vi "InjA-Image-FPGA.vi"() -> ()   [LabVIEW 2016]
uses:
  Common-Control/Glassman Readback.ctl
  Common-Control/Gate Valve Readback.ctl
  Common-Control/Faraday Cup Readback.ctl
  Common-Control/Aperture Readback.ctl
  Common-Control/Glassman Control.ctl
  <vilib>/LabVIEW Targets/FPGA/cRIO/shared/nicrio_ModuleControls/nicrio_cRIO-9871_DataBitsEnum.ctl
  <vilib>/LabVIEW Targets/FPGA/cRIO/shared/nicrio_ModuleControls/nicrio_cRIO-9871_BaudRateEnum.ctl
  <vilib>/LabVIEW Targets/FPGA/cRIO/shared/nicrio_ModuleControls/nicrio_cRIO-9871_ParityEnum.ctl
  <vilib>/LabVIEW Targets/FPGA/cRIO/shared/nicrio_ModuleControls/nicrio_cRIO-9871_StopBitsEnum.ctl
  <vilib>/Platform/TimedLoop/XDataNode/timing_clust.ctl
  <vilib>/Platform/TimedLoop/XDataNode/nitl_modes.ctl
  <vilib>/Platform/TimedLoop/XDataNode/wakeup.ctl
  <vilib>/rvi/FXPMathLib/basic elements/FxpIntAccumulator/subVIs/nifxpmath_IntAccumulator_SimConfig.ctl
  <vilib>/rvi/Emulation/niFpgaGetClockAttributes.vi
  <vilib>/rvi/Emulation/niFpgaSctlEmulationGetInTimedLoop.vi
  <vilib>/rvi/Emulation/niFpgaEmulationReportErrorSimple.vi
  <vilib>/rvi/eio/common/nirviEmuTemplateMethod_errors.vi
  <vilib>/rvi/Emulation/niFpgaCriticalErrorInLSC.vi
  <vilib>/rvi/Analysis/common/codeGenErrors/XNode/niFpgaXNodeCodeGenErrorHandle.vi
  <vilib>/rvi/FXPMathLib/basic elements/FxpIntAccumulator/simVIs/DllFxpIntAccumulator_sub.vi
  <vilib>/rvi/eio/common/nirviEmuTemplatePropertySet_errors.vi
  <vilib>/eio/EIONode/EIONode.xnode
  <vilib>/rvi/Analysis/measure/dc-rms/XNode/niFpgaDC-RMS.xnode
  <vilib>/Platform/TimedLoop/XDataNode/XDataNode.xnode
  <vilib>/rvi/FXPMathLib/basic elements/FxpIntAccumulator/XNode/nifxpmath_IntAccumulator.xnode
  <vilib>/rvi/FXPMathLib/FxpMul/XNode/nifxpmath_Multiplier.xnode
  <vilib>/eio/EIOPropertyNode/EIOPropertyNode.xnode
  <vilib>/eio/EIOMethodNode/EIOMethodNode.xnode
  <vilib>/Platform/TimedLoop/XDataNode/XDNodeRunTimeDep.lvlib
  <vilib>/rvi/FXPMathLib/sim/FxpSim.dll
  <vilib>/rvi/eio/common/nirviEmuTemplatePropertyGet_errors.vi
  <vilib>/rvi/eio/common/nirviEmuTemplatePropertyGet_noerrors.vi
  <vilib>/rvi/eio/common/nirviEmuTemplatePropertySet_noerrors.vi
panel:
  in  "InjectorA Vac Interlock":bool
  out "HV Readback loop":errorcluster
  out "HV control loop error":errorcluster
  in  "Einzel V set":T1
  in  "Pre-Acc V set":T1
  in  "Y- Steerer V set":T1
  in  "X- Steerer V set":T1
  in  "Y+ Steerer V set":T1
  in  "X+ Steerer V set":T1
  out "1st stage temp":u8[](array[numeric])
  out "Cryo status":u8[](array[numeric])
  out "2nd stage temp":u8[](array[numeric])
  out "Cryo On-time":u8[](array[numeric])
  out "Time since repurge":u8[](array[numeric])
  out "Cryo pump error":errorcluster
  out "Convectron 2":u8[](array[numeric])
  out "Ion gauge 2":u8[](array[numeric])
  out "Convectron 1":u8[](array[numeric])
  out "Ion gauge 1":u8[](array[numeric])
  out "Vac readback loop error":errorcluster
  out "Injector Magnet control error":errorcluster
  out "injector mag data":u8
  out "Inj Mag HP timed out":bool
  out "Injector Mag Field read":u8[](array[numeric])
  out "Injector Hall Probe error":errorcluster
  out "Actuator-Sensor Loop error":errorcluster
  in  "Inj Image FC Actuator":bool
  in  "Inj Image Aperture Actuator":bool
  out "Inj Image Aperture Position":T2
  out "Inj Image FC Position":T3
  out "Beamline GV Status":T4
  out "Cryo Pump GV Status":T4
  in  "LowEnd Waist Vac Interlock":bool
  in  "Cryo Pump GV Actuator":bool
  in  "Beamline GV Actuator":bool
  out "Vac Interlock":bool
  in  "Vac Interlock Bypass":bool
  out "GV Interlock loop error":errorcluster
  out "Einzel Monitor":T5
  out "Pre-Acc Monitor":T5
  out "Y- Steerer Monitor":T5
  out "Y+ Steerer Monitor":T5
  out "X- Steerer Monitor":T5
  out "X+ Steerer Monitor":T5
  in  "RT error":bool
  in  "Inj Magnet Reset":bool
  in  "Injector Magnet Set":u8[](array[numeric])=[0, 0, 0, 0, 0, 0, 0, 0, 0, 0]
  # "skipped"
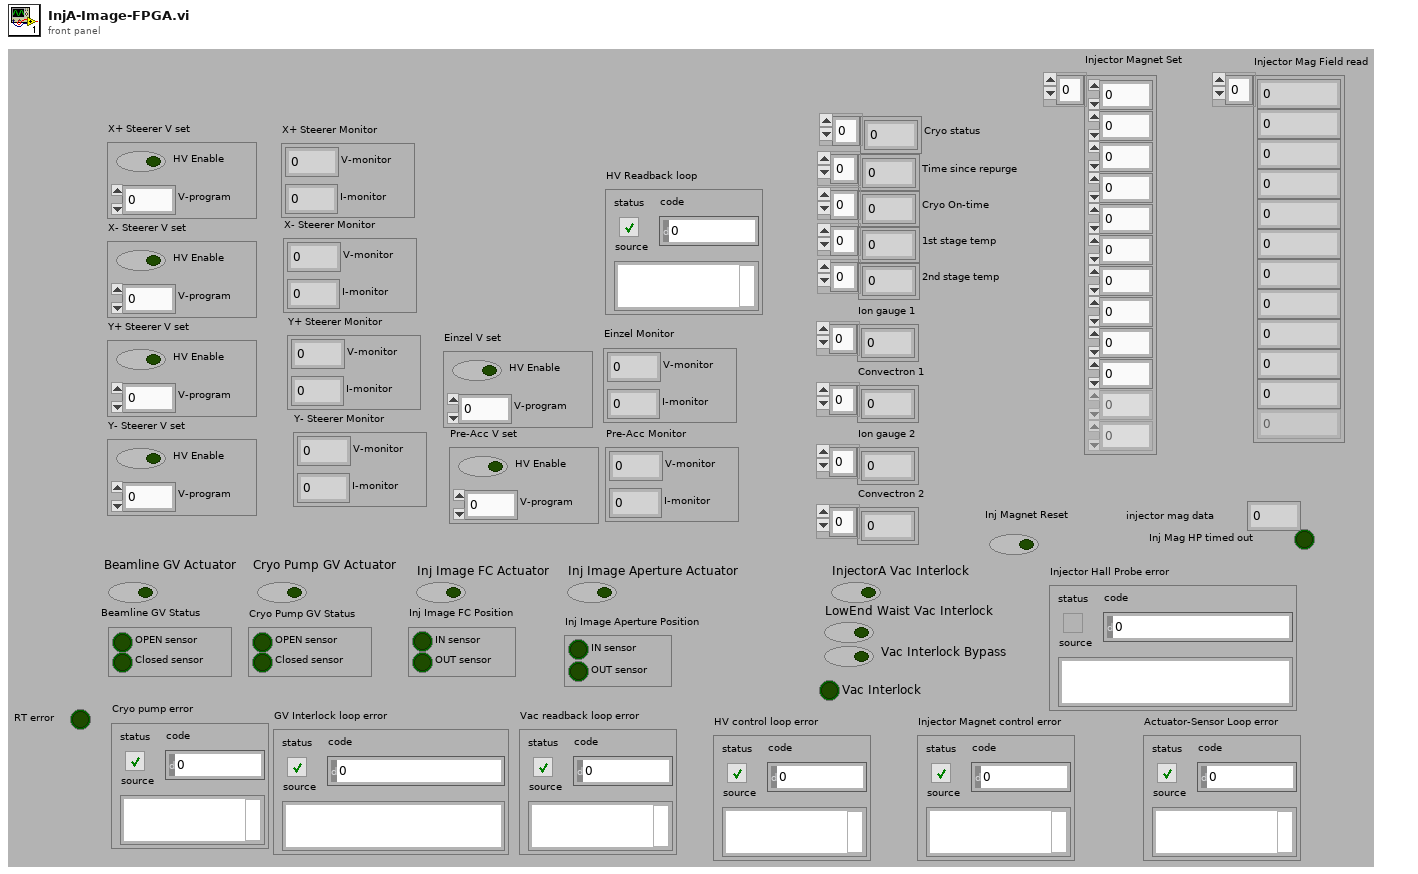
[diagram p1: front panel]
types:
  T1 = typedef "Glassman Control.ctl" = cluster{"V-program":fxp<+/-,16,5>, "HV Enable":bool}
  T2 = typedef "Aperture Readback.ctl" = cluster{"IN sensor":bool, "OUT sensor":bool}
  T3 = typedef "Faraday Cup Readback.ctl" = cluster{"IN sensor":bool, "OUT sensor":bool}
  T4 = typedef "Gate Valve Readback.ctl" = cluster{"OPEN sensor":bool, "Closed sensor":bool}
  T5 = typedef "Glassman Readback.ctl" = cluster{"I-monitor":fxp<+/-,16,5>, "V-monitor":fxp<+/-,16,5>}
  T6 = typedef "nicrio_cRIO-9871_BaudRateEnum.ctl" = enum16{"75 bps", "110 bps", "134 bps", "150 bps", "300 bps", "600 bps", "1200 bps", "1800 bps", "2400 bps", "4800 bps", "7200 bps", "9600 bps", "14.4 kbps", "19.2 kbps", "28.8 kbps", "38.4 kbps", "57.6 kbps", "115.2 kbps", "230.4 kbps", "460.8 kbps", "921.6 kbps"}
  T7 = typedef "nicrio_cRIO-9871_DataBitsEnum.ctl" = enum8{"5", "6", "7", "8"}
  T8 = typedef "nicrio_cRIO-9871_StopBitsEnum.ctl" = enum8{"1", "1.5", "2"}
  T9 = typedef "nicrio_cRIO-9871_ParityEnum.ctl" = enum8{"None", "Odd", "Even", "Mark", "Space"}
  T10 = typedef "XDNodeRunTimeDep.lvlib/timing_clust.ctl" = cluster{"Expected End [f-1]":u64, "Actual End [f-1]":u64, "Finished Late? [f-1]":bool, "Expected End [i-1]":u64, "Actual End [i-1]":u64, "Finished Late? [i-1]":bool, "Expected Start [i]":u64, "Actual Start [i]":u64, "Expected Start [f]":u64, "Actual Start [f]":u64, "Source Name":string, "Structure Name":string, "Period":i64, "Deadline":i64, "Offset":i64, "Start":i64, "Priority":i32, "Timeout":i32, "Mode":T11, "Wakeup Reason":T12, "Error":errorcluster, "Source Type":string, "Secondary Source Type":string, "Global End Time":u64, "Global Start Time":u64, "Frame Duration":u64, "Iteration Duration":u64, "Assigned CPU":i32, "I/O Scan Engine Mode":u32}
  T11 = typedef "XDNodeRunTimeDep.lvlib/nitl_modes.ctl" = enum32{"No Change", "Process missed periods, maintain original phase", "Discard missed periods, maintain original phase", "Process missed periods, ignore original phase", "Discard missed periods, ignore original phase"}
  T12 = typedef "XDNodeRunTimeDep.lvlib/wakeup.ctl" = enum32{"Normal", "Aborted", "Asynchronous wakeup", "Timing source error", "Timed loop error", "Timeout"}
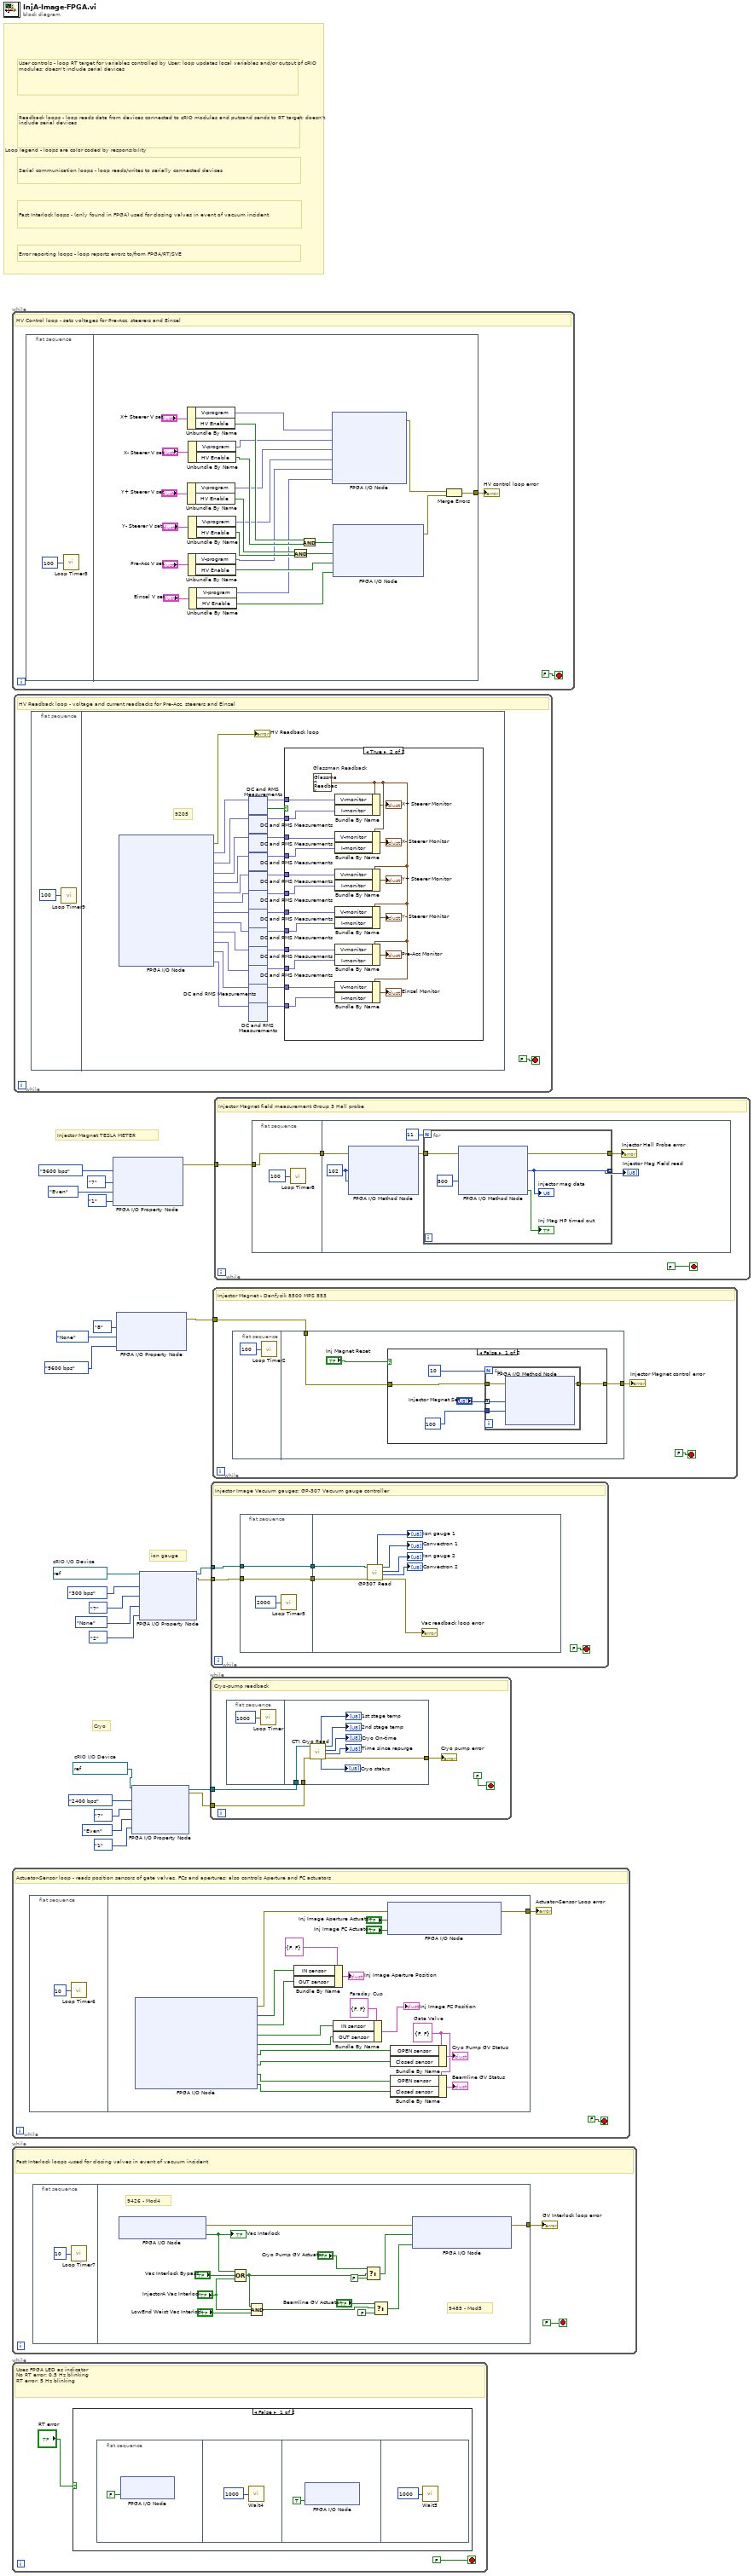
[diagram p0: block diagram]
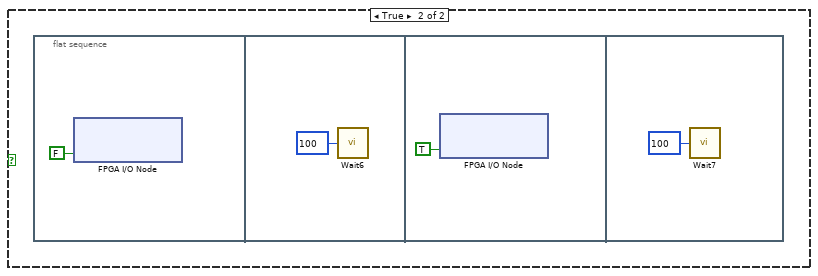
[diagram p2: hidden frame]
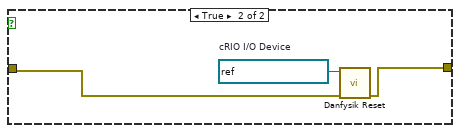
[diagram p4: hidden frame]
diagram:
  w7 = refnum<k21> "Mod7\\Port4"  # cRIO I/O Device
  w14 = refnum<k21> "Mod7\\Port3"  # cRIO I/O Device
  # "Injector Magnet TESLA METER"
  # "Fast Interlock loops - (only found in FPGA) used for closing valves in event of vacuum incident"
  # "Error reporting loops - loop reports errors to/from FPGA/RT/SVE"
  # "Serial communication loops - loop reads/writes to serially connected devices"
  # "Readback loops - loop reads data from devices connected to cRIO modules and putsand sends to RT target; doesn't include serial devices"
  # "User controls - loop RT target for variables controlled by User; loop updates local variables and/or output of cRIO modules; doesn't include serial devices"
  # "Loop legend - loops are color coded by responsibility"
  # "Cryo"
  # "ion gauge"
  n1 = while {
    stop <- FALSE stop-if-true
    # "HV Control loop - sets voltages for Pre-Acc, steerers and Einzel"
    n2 = flat-sequence {
      tunnel: [w27] -> w24
      frame #0 {
        n3 = call "Loop Timer3"("Count(mSec)"=u32 100) -> ()  [unwired: 1 out]
      }
      frame #1 {
        n4 = Unbundle By Name("X+ Steerer V set") -> ("V-program"=w35:fxp<+/-,16,5>, "HV Enable"=w36:bool)
        n5 = Unbundle By Name("Y+ Steerer V set") -> ("V-program"=w33:fxp<+/-,16,5>, "HV Enable"=w38:bool)
        n6 = Unbundle By Name("Pre-Acc V set") -> ("V-program"=w31:fxp<+/-,16,5>, "HV Enable"=w42:bool)
        n7 = Unbundle By Name("X- Steerer V set") -> ("V-program"=w34:fxp<+/-,16,5>, "HV Enable"=w37:bool)
        n8 = Unbundle By Name("Y- Steerer V set") -> ("V-program"=w32:fxp<+/-,16,5>, "HV Enable"=w39:bool)
        n9 = Unbundle By Name("Einzel V set") -> ("V-program"=w30:fxp<+/-,16,5>, "HV Enable"=w43:bool)
        n10 = And(x=w38, y=w39) -> (x .and. y?=w40:bool)
        n11 = And(x=w36, y=w37) -> (x .and. y?=w41:bool)
        n12 = xnode "FPGA I/O Node"("X+ Steerer V set"=w35, "X- Steerer V set"=w34, "Y+ Steerer V set"=w33, "Y- Steerer V set"=w32, "Pre-Acc V set"=w31, "Einzel V set"=w30) -> ("error out"=w28:errorcluster)  [unwired: 7 in, 6 out]
        n13 = xnode "FPGA I/O Node"("X Steerers HV Enable"=w41, "Y Steerers HV Enable"=w40, "Pre-Acc HV Enable"=w42, "Einzel HV Enable"=w43) -> ("error out"=w29:errorcluster)  [unwired: 5 in, 4 out]
        n14 = Merge Errors(w28, w29) -> (w27:errorcluster)
      }
    }
    "HV control loop error" <- w24
  }
  n15 = while {
    stop <- FALSE stop-if-true
    # "Actuator-Sensor loop - reads position sensors of gate valves, FCs and apertures; also controls Aperture and FC actuators"
    n16 = flat-sequence {
      tunnel: [w53] -> w50
      frame #0 {
        n17 = call "Loop Timer6"("Count(uSec)"=u32 10 ("Count(Ticks)")) -> ()  [unwired: 1 out]
      }
      frame #1 {
        w63 = T3 {"IN sensor"=FALSE, "OUT sensor"=FALSE}  # Faraday Cup
        w69 = T4 {"OPEN sensor"=FALSE, "Closed sensor"=FALSE}  # Gate Valve
        n18 = xnode "FPGA I/O Node"() -> ("error out"=w71:errorcluster, "Inj Image Aperture IN sensor"=w58:bool, "Inj Image Aperture OUT sensor"=w59:bool, "Inj Image FC IN sensor"=w60:bool, "Inj Image FC OUT sensor"=w61:bool, "Cryo Pump GV OPEN sensor"=w67:bool, "Cryo Pump GV CLOSED sensor"=w66:bool, "Beamline GV OPEN sensor"=w65:bool, "Beamline GV CLOSED sensor"=w64:bool)  [unwired: 9 in, 8 out]
        n19 = Bundle By Name(cluster=T2 {"IN sensor"=FALSE, "OUT sensor"=FALSE} ("Aperture"), "IN sensor"=w58, "OUT sensor"=w59) -> (→"Inj Image Aperture Position":T2)
        n20 = Bundle By Name(cluster=w63, "IN sensor"=w60, "OUT sensor"=w61) -> (→"Inj Image FC Position":T3)
        n21 = xnode "FPGA I/O Node"("error in"=w71, "Inj Image Aperture Actuator"="Inj Image Aperture Actuator", "Inj Image FC Actuator"="Inj Image FC Actuator") -> ("error out"=w53:errorcluster)  [unwired: 2 in, 2 out]
        n22 = Bundle By Name(cluster=w69, "OPEN sensor"=w67, "Closed sensor"=w66) -> (→"Cryo Pump GV Status":T4)
        n23 = Bundle By Name(cluster=w69, "OPEN sensor"=w65, "Closed sensor"=w64) -> (→"Beamline GV Status":T4)
      }
    }
    "Actuator-Sensor Loop error" <- w50
  }
  n24 = while {
    stop <- FALSE stop-if-true
    # "Fast Interlock loops -used for closing valves in event of vacuum incident"
    n25 = flat-sequence {
      tunnel: [w85] -> w72
      frame #0 {
        n26 = call "Loop Timer7"("Count(uSec)"=u32 10) -> ()  [unwired: 1 out]
      }
      frame #1 {
        # "9485 - Mod5"
        # "9426 - Mod4"
        n27 = xnode "FPGA I/O Node"() -> ("error out"=w87:errorcluster, "Vac Gauge Interlock"=w86:bool)  [unwired: 2 in, 1 out]
        "Vac Interlock" <- w86
        n28 = Compound Arithmetic op=OR(w86, "Vac Interlock Bypass", "InjectorA Vac Interlock") -> (w77:bool)
        n29 = Compound Arithmetic op=AND(w77, "InjectorA Vac Interlock", "LowEnd Waist Vac Interlock") -> (w78:bool)
        n30 = Select(t="Cryo Pump GV Actuator", s=w77, f=FALSE) -> (s? t:f=w80:bool)
        n31 = Select(t="Beamline GV Actuator", s=w78, f=FALSE) -> (s? t:f=w84:bool)
        n32 = xnode "FPGA I/O Node"("error in"=w87, "Cryo Pump GV Actuator"=w80, "Beamline GV Actuator"=w84) -> ("error out"=w85:errorcluster)  [unwired: 2 in, 2 out]
      }
    }
    "GV Interlock loop error" <- w72
  }
  n33 = while {
    stop <- FALSE stop-if-true
    # "Uses FPGA LED as indicator\nNo RT error: 0.5 Hz blinking\nRT error: 5 Hz blinking"
    n34 = case shown="False" "RT error" {
      frame False {
        n35 = flat-sequence {
          frame #0 {
            n36 = xnode "FPGA I/O Node"("FPGA LED"=FALSE) -> ()  [unwired: 1 in, 1 out]
          }
          frame #1 {
            n37 = call "Wait4"("Count(mSec)"=u16 1000) -> ()  [unwired: 1 out]
          }
          frame #2 {
            n38 = xnode "FPGA I/O Node"("FPGA LED"=TRUE) -> ()  [unwired: 1 in, 1 out]
          }
          frame #3 {
            n39 = call "Wait5"("Count(mSec)"=u16 1000) -> ()  [unwired: 1 out]
          }
        }
      }
      frame True {
        n40 = flat-sequence {
          frame #0 {
            n41 = xnode "FPGA I/O Node"("FPGA LED"=FALSE) -> ()  [unwired: 1 in, 1 out]
          }
          frame #1 {
            n42 = call "Wait6"("Count(mSec)"=u16 100) -> ()  [unwired: 1 out]
          }
          frame #2 {
            n43 = xnode "FPGA I/O Node"("FPGA LED"=TRUE) -> ()  [unwired: 1 in, 1 out]
          }
          frame #3 {
            n44 = call "Wait7"("Count(mSec)"=u16 100) -> ()  [unwired: 1 out]
          }
        }
      }
    }
  }
  n45 = while {
    stop <- FALSE stop-if-true
    # "HV Readback loop - voltage and current readbacks for Pre-Acc, steerers and Einzel"
    n46 = flat-sequence {
      frame #0 {
        n47 = call "Loop Timer9"("Count(mSec)"=u32 100 ("Count(Ticks)")) -> ()  [unwired: 1 out]
      }
      frame #1 {
        # "9205"
        n48 = xnode "FPGA I/O Node"() -> ("error out"=→"HV Readback loop":errorcluster, "X+ Steerer V readback"=w125:fxp<+/-,26,5>, "X+ Steerer I readback"=w123:fxp<+/-,26,5>, "X- Steerer V readback"=w121:fxp<+/-,26,5>, "X- Steerer I readback"=w119:fxp<+/-,26,5>, "Y+ Steerer V readback"=w117:fxp<+/-,26,5>, "Y+ Steerer I readback"=w115:fxp<+/-,26,5>, "Y- Steerer V readback"=w113:fxp<+/-,26,5>, "Y- Steerer I readback"=w103:fxp<+/-,26,5>, "Pre-Acc V readback"=w102:fxp<+/-,26,5>, "Pre-Acc I readback"=w109:fxp<+/-,26,5>, "Einzel V readback"=w107:fxp<+/-,26,5>, "Einzel I readback"=w105:fxp<+/-,26,5>)  [unwired: 13 in, 12 out]
        n49 = xnode "DC and RMS Measurements"("input data"=w125) -> ("DC"=w124:fxp<+/-,26,5>, "output valid"=w126:bool)  [unwired: 1 in]
        n50 = xnode "DC and RMS Measurements"("input data"=w123) -> ("DC"=w122:fxp<+/-,26,5>)  [unwired: 1 in, 1 out]
        n51 = xnode "DC and RMS Measurements"("input data"=w121) -> ("DC"=w120:fxp<+/-,26,5>)  [unwired: 1 in, 1 out]
        n52 = xnode "DC and RMS Measurements"("input data"=w119) -> ("DC"=w118:fxp<+/-,26,5>)  [unwired: 1 in, 1 out]
        n53 = xnode "DC and RMS Measurements"("input data"=w117) -> ("DC"=w116:fxp<+/-,26,5>)  [unwired: 1 in, 1 out]
        n54 = xnode "DC and RMS Measurements"("input data"=w115) -> ("DC"=w114:fxp<+/-,26,5>)  [unwired: 1 in, 1 out]
        n55 = xnode "DC and RMS Measurements"("input data"=w113) -> ("DC"=w112:fxp<+/-,26,5>)  [unwired: 1 in, 1 out]
        n56 = xnode "DC and RMS Measurements"("input data"=w103) -> ("DC"=w111:fxp<+/-,26,5>)  [unwired: 1 in, 1 out]
        n57 = xnode "DC and RMS Measurements"("input data"=w102) -> ("DC"=w110:fxp<+/-,26,5>)  [unwired: 1 in, 1 out]
        n58 = xnode "DC and RMS Measurements"("input data"=w109) -> ("DC"=w108:fxp<+/-,26,5>)  [unwired: 1 in, 1 out]
        n59 = xnode "DC and RMS Measurements"("input data"=w107) -> ("DC"=w106:fxp<+/-,26,5>)  [unwired: 1 in, 1 out]
        n60 = xnode "DC and RMS Measurements"("input data"=w105) -> ("DC"=w104:fxp<+/-,26,5>)  [unwired: 1 in, 1 out]
        n61 = case shown="True" w126 {
          tunnel: w124 -> [_ w144]
          tunnel: w122 -> [_ w143]
          tunnel: w120 -> [_ w142]
          tunnel: w118 -> [_ w141]
          tunnel: w116 -> [_ w140]
          tunnel: w114 -> [_ w139]
          tunnel: w112 -> [_ w138]
          tunnel: w111 -> [_ w133]
          tunnel: w110 -> [_ w134]
          tunnel: w108 -> [_ w135]
          tunnel: w106 -> [_ w136]
          tunnel: w104 -> [_ w137]
          frame False {
          }
          frame True {
            w145 = T5 {"I-monitor"=0.0, "V-monitor"=0.0}  # Glassman Readback
            n62 = Bundle By Name(cluster=w145, "V-monitor"=w144, "I-monitor"=w143) -> (→"X+ Steerer Monitor":T5)
            n63 = Bundle By Name(cluster=w145, "V-monitor"=w142, "I-monitor"=w141) -> (→"X- Steerer Monitor":T5)
            n64 = Bundle By Name(cluster=w145, "V-monitor"=w140, "I-monitor"=w139) -> (→"Y+ Steerer Monitor":T5)
            n65 = Bundle By Name(cluster=w145, "V-monitor"=w138, "I-monitor"=w133) -> (→"Y- Steerer Monitor":T5)
            n66 = Bundle By Name(cluster=w145, "V-monitor"=w134, "I-monitor"=w135) -> (→"Pre-Acc Monitor":T5)
            n67 = Bundle By Name(cluster=w145, "V-monitor"=w136, "I-monitor"=w137) -> (→"Einzel Monitor":T5)
          }
        }
      }
    }
  }
  n68 = xnode "FPGA I/O Property Node"("Baud Rate"=nicrio_cRIO-9871_BaudRateEnum."9600 bps", "Data Bits"=nicrio_cRIO-9871_DataBitsEnum."7", "Parity"=nicrio_cRIO-9871_ParityEnum."Even", "Stop Bits"=nicrio_cRIO-9871_StopBitsEnum."1") -> ("error out"=w20:errorcluster)  [unwired: 2 in, 1 out]
  n69 = xnode "FPGA I/O Property Node"("Data Bits"=nicrio_cRIO-9871_DataBitsEnum."8", "Parity"=nicrio_cRIO-9871_ParityEnum."None", "Baud Rate"=nicrio_cRIO-9871_BaudRateEnum."9600 bps") -> ("error out"=w15:errorcluster)  [unwired: 2 in, 1 out]
  n70 = xnode "FPGA I/O Property Node"("FPGA I/O In"=w7, "Baud Rate"=nicrio_cRIO-9871_BaudRateEnum."2400 bps", "Data Bits"=nicrio_cRIO-9871_DataBitsEnum."7", "Parity"=nicrio_cRIO-9871_ParityEnum."Even", "Stop Bits"=nicrio_cRIO-9871_StopBitsEnum."1") -> ("error out"=w6:errorcluster, "FPGA I/O Out"=w5:refnum<k21>)  [unwired: 1 in]
  n71 = xnode "FPGA I/O Property Node"("FPGA I/O In"=w14, "Baud Rate"=nicrio_cRIO-9871_BaudRateEnum."300 bps", "Data Bits"=nicrio_cRIO-9871_DataBitsEnum."7", "Parity"=nicrio_cRIO-9871_ParityEnum."None", "Stop Bits"=nicrio_cRIO-9871_StopBitsEnum."2") -> ("error out"=w9:errorcluster, "FPGA I/O Out"=w8:refnum<k21>)  [unwired: 1 in]
  n72 = while {
    tunnel: w6 -> [w1108]
    tunnel: w5 -> [w1106]
    stop <- FALSE stop-if-true
    # "Cryo-pump readback"
    n73 = flat-sequence {
      tunnel: w1108 -> [w1118]
      tunnel: [w1117] -> w1107
      tunnel: w1106 -> [w1116]
      frame #0 {
        n74 = call "Loop Timer"("Count(mSec)"=u32 1000) -> ()  [unwired: 1 out]
      }
      frame #1 {
        n75 = call "CTI Cryo Read.vi"("error in (no error)"=w1118, "cRIO I/O Device"=w1116) -> ("error out"=w1117:errorcluster, "Time since repurge"=→"Time since repurge":u8[], "Cryo On-time"=→"Cryo On-time":u8[], "2nd stage temp"=→"2nd stage temp":u8[], "Cryo status"=→"Cryo status":u8[], "1st stage temp"=→"1st stage temp":u8[])  [unwired: 4 in]
      }
    }
    "Cryo pump error" <- w1107
  }
  n76 = while {
    tunnel: w9 -> [w1122]
    tunnel: w8 -> [w1121]
    stop <- FALSE stop-if-true
    # "Injector Image Vacuum gauges: GP-307 Vacuum gauge controller"
    n77 = flat-sequence {
      tunnel: w1121 -> [w1125]
      tunnel: w1122 -> [w1126]
      tunnel: [w1126] -> w1120
      tunnel: [w1125] -> w1119
      tunnel: w1120 -> [w1128]
      tunnel: w1119 -> [w1127]
      frame #0 {
        n78 = call "Loop Timer5"("Count(mSec)"=u32 2000 ("Count(Ticks)")) -> ()  [unwired: 1 out]
      }
      frame #1 {
        n79 = call "GP307 Read.vi"("error in"=w1128, "cRIO I/O Device"=w1127) -> ("error out"=→"Vac readback loop error":errorcluster, "Convectron 2"=→"Convectron 2":u8[], "Ion gauge 2"=→"Ion gauge 2":u8[], "Convectron 1"=→"Convectron 1":u8[], "Ion gauge 1"=→"Ion gauge 1":u8[])  [unwired: 5 in]
      }
    }
  }
  n80 = while {
    tunnel: w15 -> [w1135]
    stop <- FALSE stop-if-true
    # "Injector Magnet - Danfysik 8500 MPS 853"
    n81 = flat-sequence {
      tunnel: w1135 -> [w1139]
      tunnel: [w1138] -> w1134
      frame #0 {
        n82 = call "Loop Timer2"("Count(mSec)"=u32 100) -> ()  [unwired: 1 out]
      }
      frame #1 {
        n83 = case shown="False" "Inj Magnet Reset" {
          tunnel: w1139 -> [w1141 w1150]
          tunnel: [w1142 w1151] -> w1138
          frame False {
            n84 = for {
              N: 10 -> [_]
              tunnel: 100 ("Timeout (ms)") -> [w1149]
              tunnel: "Injector Magnet Set" -> [w1148] mode=indexing
              tunnel: w1141 -> [w1147]
              tunnel: [w1146] -> w1142
              n85 = xnode "FPGA I/O Method Node"("error in"=w1147, "Data"=w1148, "Timeout (ms)"=w1149) -> ("error out"=w1146:errorcluster)  [unwired: 1 in, 2 out]
            }
          }
          frame True {
            w1152 = refnum<k21> "Mod7\\Port2"  # cRIO I/O Device
            n86 = call "Danfysik Reset.vi"("error in"=w1150, "cRIO I/O Device"=w1152) -> ("error out"=w1151:errorcluster)  [unwired: 9 in]
          }
        }
      }
    }
    "Injector Magnet control error" <- w1134
  }
  n87 = while {
    tunnel: w20 -> [w1154]
    stop <- FALSE stop-if-true
    # "Injector Magnet field measurement Group 3 Hall probe"
    n88 = flat-sequence {
      tunnel: w1154 -> [w1156]
      tunnel: [w1156] -> w1153
      tunnel: w1153 -> [w1158]
      frame #0 {
        n89 = call "Loop Timer8"("Count(mSec)"=u32 100) -> ()  [unwired: 1 out]
      }
      frame #1 {
        w1162 = u8 102 ("Data")
        n90 = xnode "FPGA I/O Method Node"("error in"=w1158, "Data"=w1162, "Timeout (ms)"=w1162) -> ("error out"=w1161:errorcluster)  [unwired: 1 in, 2 out]
        n91 = for {
          N: 11 ("Numeric 3") -> [_]
          tunnel: [w1166] -> w1159 mode=indexing
          tunnel: w1161 -> [w1165]
          tunnel: [w1164] -> w1160
          n92 = xnode "FPGA I/O Method Node"("error in"=w1165, "Timeout (ms)"=500) -> ("error out"=w1164:errorcluster, "Data"=w1166:u8, "Timed Out"=→"Inj Mag HP timed out":bool)  [unwired: 1 in, 1 out]
          "injector mag data" <- w1166
        }
        "Injector Mag Field read" <- w1159
        "Injector Hall Probe error" <- w1160
      }
    }
  }
